vi "177-MalformedXmlAttribute.vi"(8 "error in":errorcluster) -> (0 "error out":errorcluster)   [LabVIEW 2020]
uses:
  classes/MsgSerializer.XML/MsgSerializer.XML.lvclass
  classes/MsgSerializer.XML/format -- enum.ctl
  classes/MsgSerializer.XML/MsgSerializer.XML.lvclass/MsgSerializer.XML.ctl
  classes/Properties.Assert/Properties.Assert.lvclass
  C:/projects/caraya/src/classes/Properties/Properties.lvclass
  classes/Assert/Assert Equal Value_Variant.vi
  classes/Test/Test.lvclass
  classes/Assert/Assert.lvclass
  classes/Properties/Properties.lvclass
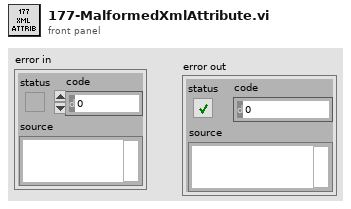
[diagram p1: front panel]
types:
  T1 = typedef "Caraya.lvlib/MsgSerializer.XML.lvclass/format -- enum.ctl" = enum16{"value", "tag", "property"}
  T2 = cluster{"Label (VI Title)":string, "Label (VI Title)":string}
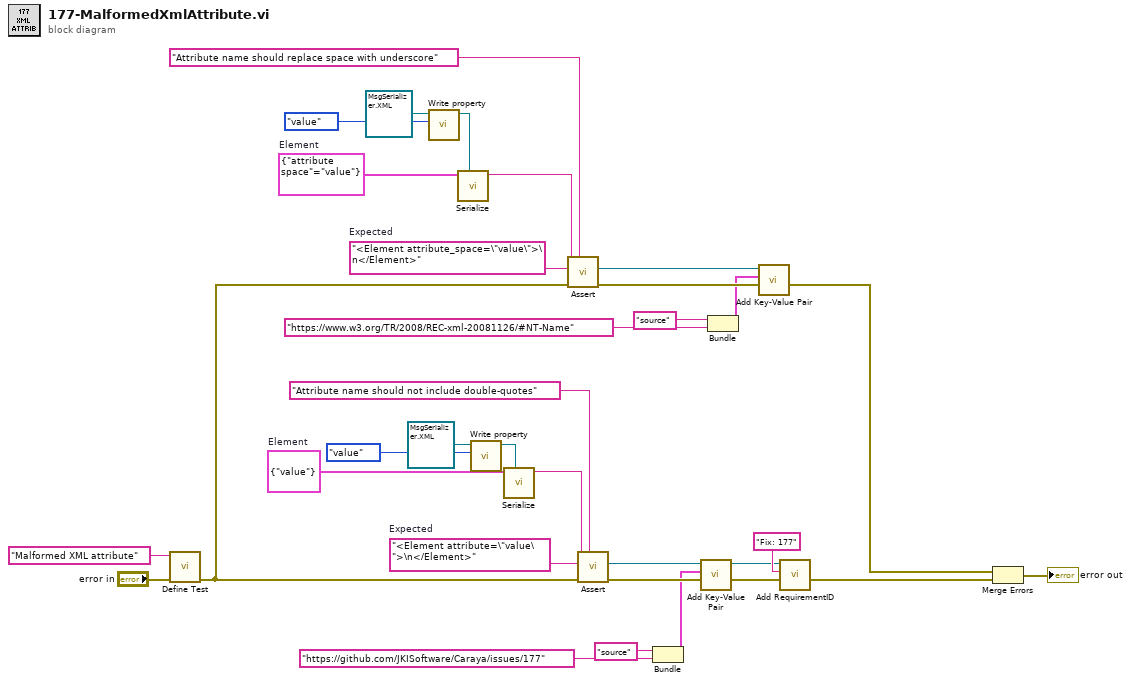
[diagram p0: block diagram]
diagram:
  w22 = "<Element attribute_space=\"value\">\n</Element>"  # Expected
  w28 = cluster{"attribute space":string} {"attribute space"="value"}  # Element
  w29 = "<Element attribute=\"value\">\n</Element>"  # Expected
  w31 = cluster{"attribute":string} {"attribute"="value"}  # Element
  n1 = call "Define Test.vi"("error in (no error)"="error in", "Label (VI Title)"="Malformed XML attribute") -> ("error out"=w18:errorcluster)  [unwired: 8 in, 1 out]
  n2 = call "Write property.vi"("format"=format_--_enum."value", "MsgSerializer.XMLProperty in"=refnum<class "MsgSerializer.XML.lvclass"> refnum ("Caraya.lvlib:MsgSerializer.XML.lvclass")) -> ("MsgSerializer.XMLProperty out"=w25:refnum<class "MsgSerializer.XML.lvclass">)  [unwired: 9 in]
  n3 = call-dynamic "Serialize.vi"("MsgSerializer"=w25, "Value"=w28) -> ("Serialized Message"=w17:string)  [unwired: 8 in, 1 out]
  n4 = call "Write property.vi"("format"=format_--_enum."value", "MsgSerializer.XMLProperty in"=refnum<class "MsgSerializer.XML.lvclass"> refnum ("Caraya.lvlib:MsgSerializer.XML.lvclass")) -> ("MsgSerializer.XMLProperty out"=w19:refnum<class "MsgSerializer.XML.lvclass">)  [unwired: 9 in]
  n5 = call-dynamic "Serialize.vi"("MsgSerializer"=w19, "Value"=w31) -> ("Serialized Message"=w30:string)  [unwired: 8 in, 1 out]
  n6 = call-poly "Assert.vi"("Label"="Attribute name should replace space with underscore" ("Label (VI Title)"), "error in (no error)"=w18, "Y"=w22, "X"=w17) -> ("error out"=w16:errorcluster, "Properties.Assert"=w12:refnum<class "Properties.Assert.lvclass">)  [unwired: 6 in]
  n7 = call-poly "Assert.vi"("Label"="Attribute name should not include double-quotes" ("Label (VI Title)"), "error in (no error)"=w18, "Y"=w29, "X"=w30) -> ("error out"=w3:errorcluster, "Properties.Assert"=w5:refnum<class "Properties.Assert.lvclass">)  [unwired: 6 in]
  n8 = Bundle("Label (VI Title)"="source", "Label (VI Title)"="https://github.com/JKISoftware/Caraya/issues/177") -> (w1:T2)  [unwired: 1 in]
  n9 = call "Add Key-Value Pair.vi"("error in (no error)"=w3, "entry"=w1, "Properties in"=w5) -> ("error out"=w2:errorcluster, "Properties out"=w4:refnum<class "Properties.Assert.lvclass">)  [unwired: 7 in]
  n10 = Bundle("Label (VI Title)"="source", "Label (VI Title)"="https://www.w3.org/TR/2008/REC-xml-20081126/#NT-Name") -> (w14:T2)  [unwired: 1 in]
  n11 = call "Add Key-Value Pair.vi"("error in (no error)"=w16, "entry"=w14, "Properties in"=w12) -> ("error out"=w11:errorcluster)  [unwired: 7 in, 1 out]
  n12 = call "Add RequirementID.vi"("error in (no error)"=w2, "Requirement ID"="Fix: 177", "Properties"=w4) -> ("error out"=w9:errorcluster)  [unwired: 7 in, 1 out]
  n13 = Merge Errors(w11, w9) -> (→"error out":errorcluster)
